vi "Micrometer Heading v2.vi"() -> ()   [LabVIEW 2024]
uses:
  <vilib>/Utility/miscctls.llb/LVRowAndColumnTypeDef.ctl
  Library/Class/Renishaw-XL80_EMU/Renishaw-XL80_EMU.lvclass
  Library/Class/Renishaw-XL80/Renishaw-XL80.lvclass
  <vilib>/Utility/file.llb/Write Delimited Spreadsheet (string).vi
  <vilib>/Analysis/1siggen.llb/Ramp Pattern by Delta.vi
  <vilib>/Analysis/NI_AALBase.lvlib
panel:
  in  "Table Control Periodic":string[][](table)
  in  "Range":u16(ring)=10 caption="mm/inch" items=["0-25"=10, "0-50"=20]
  out "Periodic Range of Errors":dbl=nan format="%#.8f"
  out "Progressive Range of Errors":dbl=nan format="%#.8f"
  out "error out 2":errorcluster
  in  "Clear Result":bool
  in  "Export to CSV":bool
  in  "Delete Down":bool
  in  "Read Down":bool
  in  "Delete Up":bool
  out "Down Values":dbl[](array[numeric]) caption="Down Value" format="%#.6f"
  in  "Read Up":bool
  out "Backlash":dbl=nan format="%#.8f"
  out "Repeatability":dbl=nan format="%#.8f"
  in  "Calculate Read":bool
  out "Up Values":dbl[](array[numeric]) caption="Up Value" format="%#.6f"
  in  "Nominal":dbl caption="Job No." format="%#.8f"
  out "output cluster":cluster{"nextRow":dbl, "nextColumn":dbl}
  out "Current":T1
  out "ScanCode":i16
  in  "Table Control Progressive":string[][](table)
  out "Signal":dbl(slide) scale=0.0..31.0
  in  "sign_mode":bool
  out "Zero Value":dbl format="%_8f"
  out "Mat Temp":dbl[](array[numeric]) caption="Mat Temp(°C)"
  out "Air Temp":dbl caption="Air Temp(°C)"
  in  "Reset":bool
  in  "Connect":bool
  in  "Zero":bool
  out "Serial Number":string caption="Laser Device ID"
  out "Connected":bool
  in  "Precision":u16(ring)=4 items=["0 digit", "1 digit", "2 digits", "3 digits", "4 digits", "5 digits", "6 digits"]
  in  "Unit":u16(ring) caption="mm/inch" items=["mm", "inch"]
  out "Measurement":dbl format="%.4f"
  in  "Description":string
  in  "Manufacturer":string
  in  "Ref equipment ID":string
  in  "Model No.":string
  in  "S/No. or ID":string
  in  "Job No.":string
  out "uncalibrated":dbl
  out "error out":errorcluster
  in  "error IO":errorcluster
  # "Read Value"
  # "Repeatability & Backlash"
  # "Job Info"
  # "DUT Info"
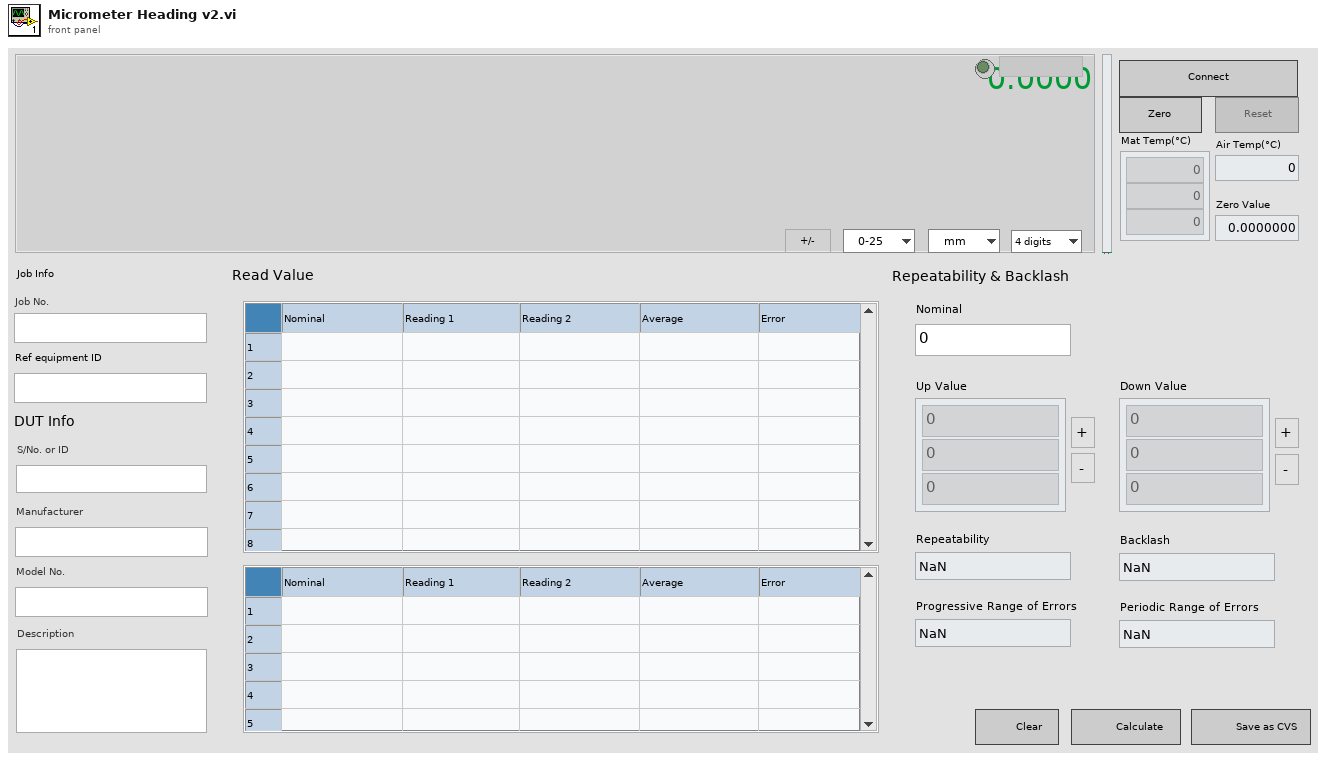
[diagram p1: front panel]
types:
  T1 = typedef "LVRowAndColumnTypeDef.ctl" = cluster{"Row":i32, "Column":i32}
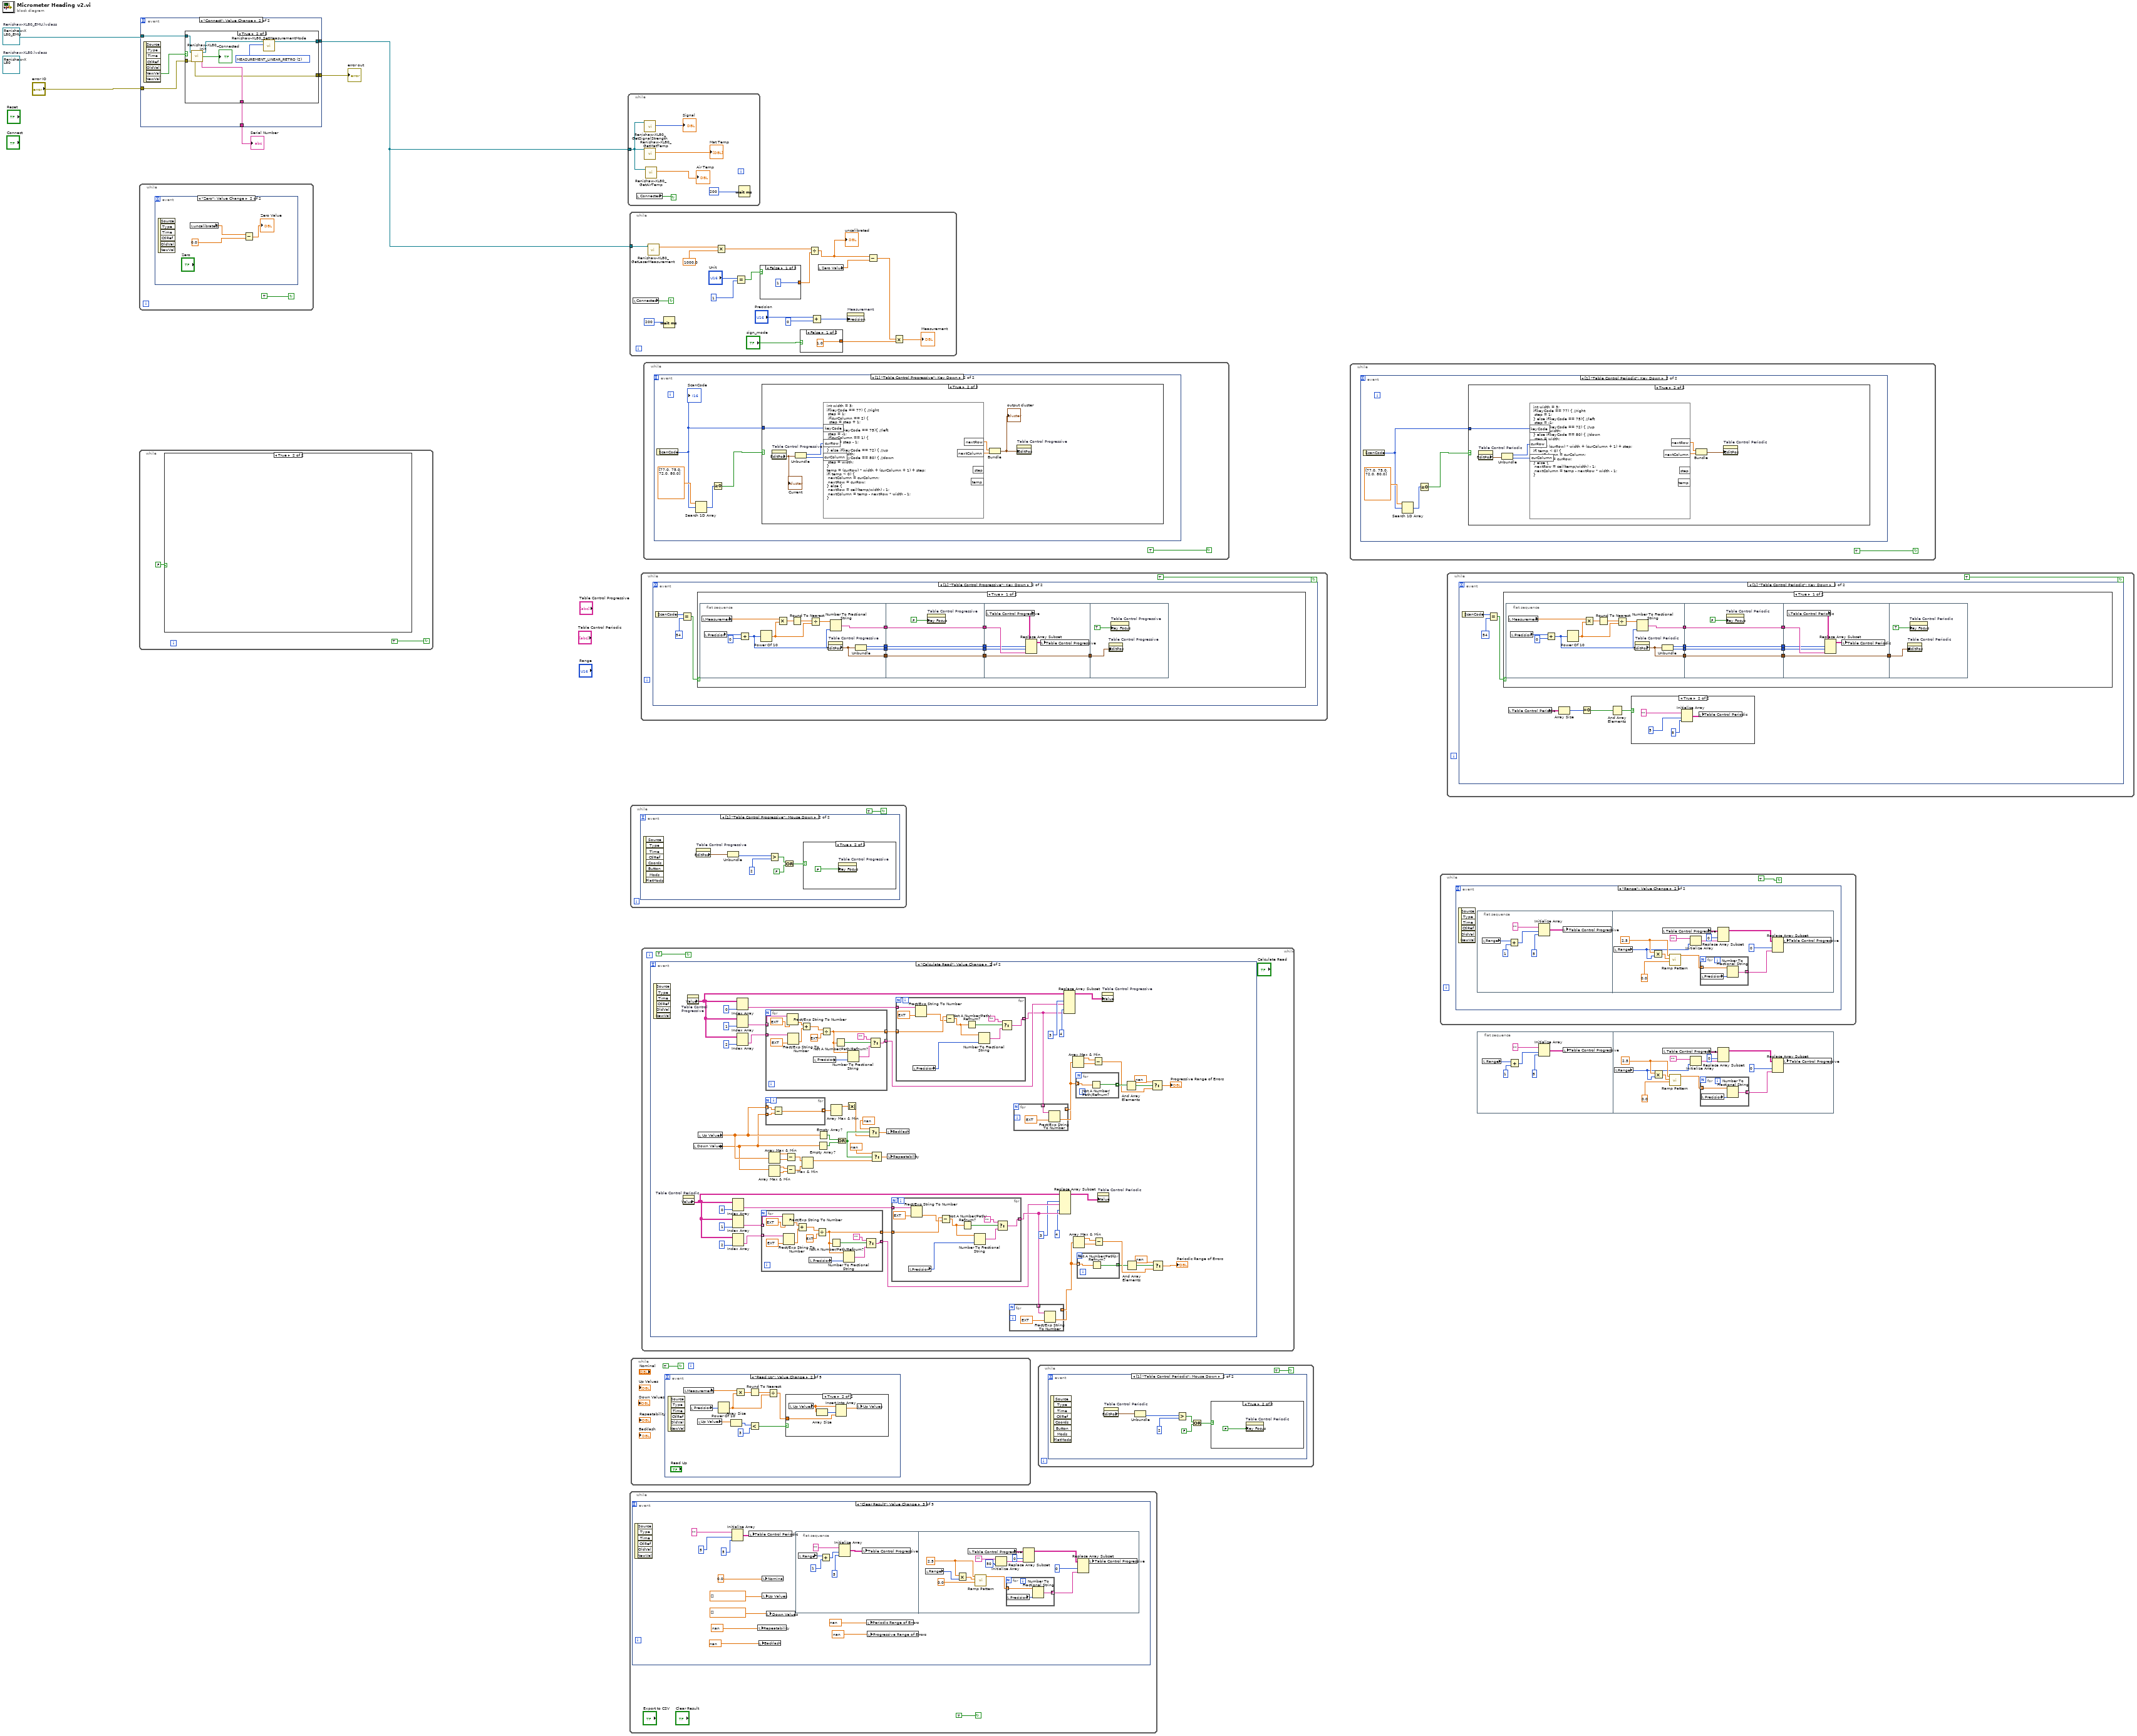
[diagram p0: block diagram]
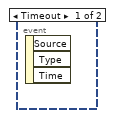
[diagram p2: hidden frame]
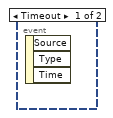
[diagram p4: hidden frame]
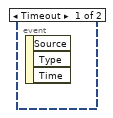
[diagram p6: hidden frame]
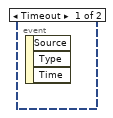
[diagram p9: hidden frame]
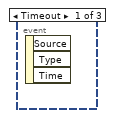
[diagram p10: hidden frame]
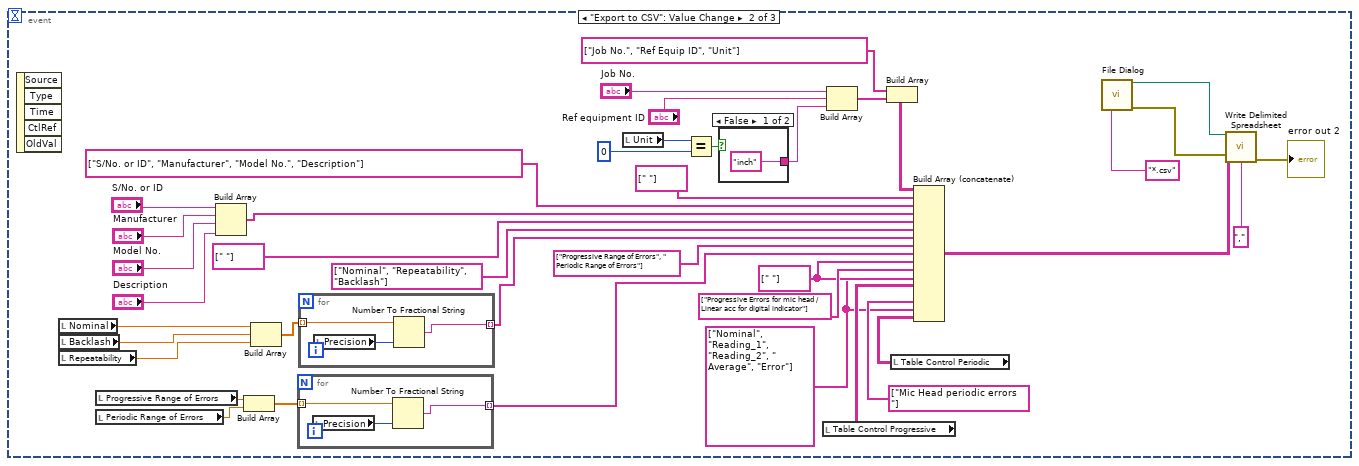
[diagram p11: hidden frame]
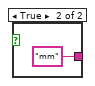
[diagram p12: hidden frame]
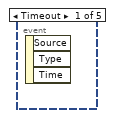
[diagram p13: hidden frame]
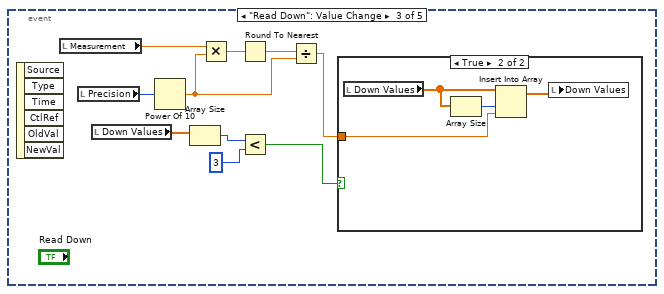
[diagram p15: hidden frame]
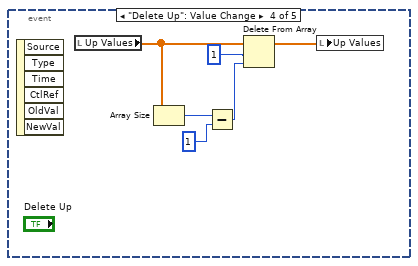
[diagram p17: hidden frame]
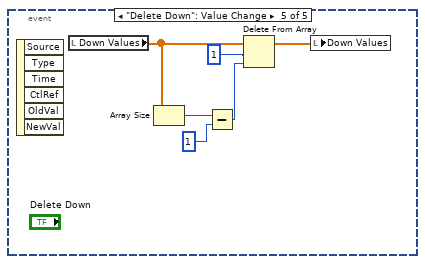
[diagram p18: hidden frame]
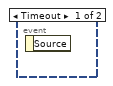
[diagram p19: hidden frame]
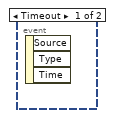
[diagram p20: hidden frame]
diagram:
  w1 = refnum<class "Renishaw-XL80_EMU.lvclass"> refnum  # Renishaw-XL80_EMU.lvclass
  (unwired) refnum<class "Renishaw-XL80.lvclass"> refnum  # Renishaw-XL80.lvclass
  n1 = while {
    stop <- TRUE continue-if-true
    n2 = case shown="True" FALSE {
      frame False {
      }
      frame True {
      }
    }
  }
  n3 = while {
    stop <- TRUE continue-if-true
    n4 = event shown="[1] \"Zero\": Value Change" {
      selector: _ -> [_ _]
      dyn-events: _ -> [_ _]
      timeout: _ -> [_ _]
      event Timeout {
        n5 = event-data() -> ()  [unwired: 1 in, 3 out]
      }
      event "Zero": Value Change {
        n6 = event-data() -> ()  [unwired: 1 in, 6 out]
        n7 = local read "uncalibrated"() -> (w11:dbl)
        n8 = Subtract(x=w11, y=0.0) -> (x-y=→"Zero Value":dbl)
      }
    }
  }
  n9 = event shown="[1] \"Connect\": Value Change" {
    selector: _ -> [_ _]
    dyn-events: _ -> [_ _]
    timeout: _ -> [_ _]
    tunnel: w1 -> [_ w17]
    tunnel: [_ w16] -> w4
    tunnel: [_ w15] -> w5
    tunnel: "error IO" -> [_ w14]
    tunnel: [_ w13] -> w3
    event Timeout {
      n10 = event-data() -> ()  [unwired: 1 in, 3 out]
    }
    event "Connect": Value Change {
      n11 = event-data() -> ("NewVal"=w12:bool)  [unwired: 1 in, 6 out]
      n12 = case shown="True" w12 {
        tunnel: w17 -> [w22 w30]
        tunnel: ["N/A" ("Serial Number") w29] -> w15
        tunnel: [w21 w24] -> w16
        tunnel: w14 -> [w20 w28]
        tunnel: [w19 w27] -> w13
        frame False {
          n13 = call-dynamic "Renishaw-XL80_Close.vi"("error in (no error)"=w20, "Renishaw-XL80_EMU in"=w22) -> ("error out"=w19:errorcluster, "Renishaw-XL80_EMU out"=w21:refnum<class "Renishaw-XL80_EMU.lvclass">)  [unwired: 8 in]
        }
        frame True {
          w23 = 2 items=["MEASUREMENT_INDETERMINATE", "MEASUREMENT_LINEAR_PLANE", "MEASUREMENT_LINEAR_RETRO", "MEASUREMENT_ANGULAR", "MEASUREMENT_STRAIGHTNESS_SHORT", "MEASUREMENT_STRAIGHTNESS_LONG", "MEASUREMENT_VELOCITY_RETRO"] ("MeasurementMode")
          n14 = call-dynamic "Renishaw-XL80_Init.vi"("error in (no error)"=w28, "Renishaw-XL80_EMU in"=w30) -> ("error out"=w27:errorcluster, "Serial Number"=w29:string, "Connect"=→"Connected":bool, "Renishaw-XL80_EMU out"=w25:refnum<class "Renishaw-XL80_EMU.lvclass">)  [unwired: 6 in]
          n15 = call-dynamic "Renishaw-XL80_SetMeasurementMode.vi"("MeasurementMode"=w23, "Renishaw-XL80_EMU in"=w25) -> ("Renishaw-XL80_EMU out"=w24:refnum<class "Renishaw-XL80_EMU.lvclass">)  [unwired: 8 in, 1 out]
        }
      }
    }
  }
  "error out" <- w3
  "Serial Number" <- w5
  n16 = while {
    tunnel: w4 -> [w32]
    stop <- w33 continue-if-true
    n17 = local read "Connected"() -> (w33:bool)
    n18 = call-dynamic "Renishaw-XL80_GetSignalStrength.vi"("Renishaw-XL80_EMU in"=w32) -> ("Signal Strength"=→"Signal":i16)  [unwired: 8 in, 2 out]
    n19 = call-dynamic "Renishaw-XL80_GetMatTemp.vi"("Renishaw-XL80_EMU in"=w32) -> ("Temperature Array"=→"Mat Temp":dbl[])  [unwired: 7 in, 3 out]
    n20 = call-dynamic "Renishaw-XL80_GetAirTemp.vi"("Renishaw-XL80_EMU in"=w32) -> ("GetAirTemp"=→"Air Temp":dbl)  [unwired: 7 in, 3 out]
    n21 = Wait (ms)(milliseconds to wait=u32 200) -> ()  [unwired: 1 out]
  }
  n22 = while {
    tunnel: w4 -> [w55]
    stop <- w44 continue-if-true
    n23 = local read "Connected"() -> (w44:bool)
    n24 = call-dynamic "Renishaw-XL80_GetLaserMeasurement.vi"("Renishaw-XL80_EMU in"=w55) -> ("GetLaserMeasurement"=w53:dbl)  [unwired: 7 in, 3 out]
    n25 = Wait (ms)(milliseconds to wait=u32 200) -> ()  [unwired: 1 out]
    n26 = Multiply(x=w53, y=1000.0) -> (x*y=w45:dbl)
    n27 = Equal?(x="Unit", y=u16 1) -> (x = y?=w47:bool)
    n28 = case shown="False" w47 {
      tunnel: [1 25.4] -> w46
      frame False {
      }
      frame True {
      }
    }
    n29 = case shown="False" "sign_mode" {
      tunnel: [1.0 -1.0] -> w39
      frame False {
      }
      frame True {
      }
    }
    n30 = Divide(x=w45, y=w46) -> (x/y=w42:dbl)
    "uncalibrated" <- w42
    n31 = Add(x="Precision", y=u16 0) -> (x+y=w41:u16)
    n32 = local read "Zero Value"() -> (w43:dbl)
    n33 = property on="Measurement" class="DigNum (strict)"("Precision"=w41) -> ()  [unwired: 2 in, 2 out]
    n34 = Subtract(x=w42, y=w43) -> (x-y=w38:dbl)
    n35 = Multiply(x=w38, y=w39) -> (x*y=→"Measurement":dbl)
  }
  n36 = while {
    stop <- TRUE continue-if-true
    n37 = event shown="[2] \"Clear Result\": Value Change" {
      selector: _ -> [_ _ _]
      dyn-events: _ -> [_ _ _]
      timeout: _ -> [_ _ _]
      event Timeout {
        n38 = event-data() -> ()  [unwired: 1 in, 3 out]
      }
      event "Export to CSV": Value Change {
        w69 = string[] [" "] ("array")
        w66 = string[] ["Nominal", "Reading_1", "Reading_2", " Average", "Error"]
        n39 = event-data() -> ()  [unwired: 1 in, 5 out]
        n40 = local read "Nominal"() -> (w71:dbl)
        n41 = local read "Backlash"() -> (w84:dbl)
        n42 = local read "Repeatability"() -> (w83:dbl)
        n43 = local read "Progressive Range of Errors"() -> (w64:dbl)
        n44 = local read "Periodic Range of Errors"() -> (w62:dbl)
        n45 = Build Array("S/No. or ID", "Manufacturer", "Model No.", "Description") -> (w73:string[])
        n46 = Build Array(w64, w62) -> (w63:dbl[])
        n47 = Build Array(w71, w84, w83) -> (w82:dbl[])
        n48 = for {
          tunnel: w63 -> [w102] mode=indexing
          tunnel: [w101] -> w61 mode=indexing
          n49 = local read "Precision"() -> (w103:u16)
          n50 = Number To Fractional String(number=w102, precision (6)=w103) -> (F-format string=w101:string)  [unwired: 2 in]
        }
        n51 = for {
          tunnel: w82 -> [w105] mode=indexing
          tunnel: [w104] -> w80 mode=indexing
          n52 = local read "Precision"() -> (w106:u16)
          n53 = Number To Fractional String(number=w105, precision (6)=w106) -> (F-format string=w104:string)  [unwired: 2 in]
        }
        n54 = local read "Unit"() -> (w93:u16)
        n55 = Equal?(x=w93, y=u16 0) -> (x = y?=w91:bool)
        n56 = case shown="False" w91 {
          tunnel: ["inch" "mm"] -> w90
          frame False {
          }
          frame True {
          }
        }
        n57 = local read "Table Control Progressive"() -> (w79:string[][])
        n58 = Build Array("Job No.", "Ref equipment ID", w90) -> (w88:string[])
        n59 = Build Array(string[] ["Job No.", "Ref Equip ID", "Unit"] ("element"), w88) -> (w87:string[][])
        n60 = local read "Table Control Periodic"() -> (w67:string[][])
        n61 = Build Array (concatenate)(w87, string[] [" "] ("array"), string[] ["S/No. or ID", "Manufacturer", "Model No.", "Description"] ("element"), w73, string[] [" "] ("array"), string[] ["Nominal", "Repeatability", "Backlash"] ("element"), w80, string[] ["Progressive Range of Errors", " Periodic Range of Errors"] ("element"), w61, w69, string[] ["Progressive Errors for mic head / Linear acc for digital indicator"] ("element"), w66, w79, w69, string[] ["Mic Head periodic errors "] ("element"), w66, w67) -> (w99:string[][])
        n62 = call "File Dialog"("pattern (all files)"="*.csv") -> ("selected path"=w98:path, "error out"=w95:errorcluster)  [unwired: 11 in, 2 out]
        n63 = call-poly <vilib>:"Write Delimited Spreadsheet.vi"("file path (dialog if empty)"=w98, "2D data"=w99, "error in (no error)"=w95, "delimiter (\\t)"="," ("delimiter (\\t)")) -> ("error out"=→"error out 2":errorcluster)  [unwired: 10 in, 1 out]
      }
      event "Clear Result": Value Change {
        n64 = event-data() -> ()  [unwired: 1 in, 6 out]
        n65 = Initialize Array("", 5 ("dimension size"), 5 ("dimension size")) -> (w119:string[][])
        n66 = local write "Table Control Periodic"(w119) -> ()
        n67 = local write "Repeatability"(nan ("Nominal")) -> ()
        n68 = local write "Backlash"(nan ("Nominal")) -> ()
        n69 = local write "Nominal"(0.0 ("Nominal")) -> ()
        n70 = local write "Up Values"(dbl[] [] ("Up Values")) -> ()
        n71 = local write "Down Values"(dbl[] [] ("Up Values")) -> ()
        n72 = flat-sequence {
          frame #0 {
            n73 = local read "Range"() -> (w121:u16)
            n74 = Add(x=w121, y=u16 1) -> (x+y=w122:u16)
            n75 = Initialize Array("", w122, 5 ("dimension size")) -> (w125:string[][])
            n76 = local write "Table Control Progressive"(w125) -> ()
          }
          frame #1 {
            w126 = 2.5 ("delta")
            n77 = local read "Range"() -> (w127:u16)
            n78 = Multiply(x=w126, y=w127) -> (x*y=w128:dbl)
            n79 = local read "Table Control Progressive"() -> (w134:string[][])
            n80 = call-poly <vilib>:"Ramp Pattern.vi"("start"=0.0, "end"=w128, "delta"=w126) -> ("Ramp Pattern"=w130:dbl[])  [unwired: 6 in, 2 out]
            n81 = Initialize Array("", 50 ("dimension size")) -> (w137:string[])
            n82 = for {
              tunnel: w130 -> [w142] mode=indexing
              tunnel: [w140] -> w132 mode=indexing
              n83 = local read "Precision"() -> (w141:u16)
              n84 = Number To Fractional String(number=w142, precision (6)=w141) -> (F-format string=w140:string)  [unwired: 2 in]
            }
            n85 = Replace Array Subset(array=w134, new element=w137, index (col)=0) -> (w139:string[][])  [unwired: 1 in]
            n86 = Replace Array Subset(array=w139, new element=w132, index (col)=0) -> (w131:string[][])  [unwired: 1 in]
            n87 = local write "Table Control Progressive"(w131) -> ()
          }
        }
        n88 = local write "Periodic Range of Errors"(nan ("Nominal")) -> ()
        n89 = local write "Progressive Range of Errors"(nan ("Nominal")) -> ()
      }
    }
  }
  n90 = while {
    stop <- TRUE continue-if-true
    n91 = event shown="[1] \"Table Control Progressive\": Mouse Down" {
      selector: _ -> [_ _]
      dyn-events: _ -> [_ _]
      timeout: _ -> [_ _]
      event Timeout {
        n92 = event-data() -> ()  [unwired: 1 in, 3 out]
      }
      event "Table Control Progressive": Mouse Down {
        n93 = event-data() -> ()  [unwired: 1 in, 8 out]
        n94 = property on="Table Control Progressive" class="Tbl (strict)"() -> ("EditPos"=w149:T1)  [unwired: 2 in, 2 out]
        n95 = Unbundle(w149) -> ("Column"=w147:i32)  [unwired: 1 out]
        n96 = Greater?(x=w147, y=2) -> (0:w146:bool)
        n97 = Or(x=w146, y=FALSE) -> (x .or. y?=w145:bool)
        n98 = case shown="True" w145 {
          frame False {
          }
          frame True {
            n99 = property on="Table Control Progressive" class="Tbl (strict)"("Key Focus"=FALSE) -> ()  [unwired: 2 in, 2 out]
          }
        }
      }
    }
  }
  n100 = while {
    stop <- TRUE continue-if-true
    n101 = event shown="[1] \"Read Up\": Value Change" {
      selector: _ -> [_ _ _ _ _]
      dyn-events: _ -> [_ _ _ _ _]
      timeout: _ -> [_ _ _ _ _]
      event Timeout {
        n102 = event-data() -> ()  [unwired: 1 in, 3 out]
      }
      event "Read Up": Value Change {
        n103 = event-data() -> ()  [unwired: 1 in, 6 out]
        n104 = local read "Measurement"() -> (w157:dbl)
        n105 = local read "Precision"() -> (w161:u16)
        n106 = local read "Up Values"() -> (w156:dbl[])
        n107 = Power Of 10(x=w161) -> (10^x=w158:dbl)
        n108 = Array Size(array=w156) -> (size(s)=w155:i32)
        n109 = Multiply(x=w157, y=w158) -> (x*y=w160:dbl)
        n110 = Round To Nearest(number=w160) -> (nearest integer value=w159:dbl)
        n111 = Less?(x=w155, y=3) -> (x < y?=w153:bool)
        n112 = Divide(x=w159, y=w158) -> (x/y=w152:dbl)
        n113 = case shown="True" w153 {
          tunnel: w152 -> [_ w165]
          frame False {
          }
          frame True {
            n114 = local read "Up Values"() -> (w164:dbl[])
            n115 = Array Size(array=w164) -> (size(s)=w163:i32)
            n116 = Insert Into Array(array=w164, index=w163, new element=w165) -> (w162:dbl[])
            n117 = local write "Up Values"(w162) -> ()
          }
        }
      }
      event "Read Down": Value Change {
        n118 = event-data() -> ()  [unwired: 1 in, 6 out]
        n119 = local read "Measurement"() -> (w171:dbl)
        n120 = local read "Precision"() -> (w175:u16)
        n121 = local read "Down Values"() -> (w170:dbl[])
        n122 = Power Of 10(x=w175) -> (10^x=w172:dbl)
        n123 = Array Size(array=w170) -> (size(s)=w169:i32)
        n124 = Multiply(x=w171, y=w172) -> (x*y=w174:dbl)
        n125 = Round To Nearest(number=w174) -> (nearest integer value=w173:dbl)
        n126 = Less?(x=w169, y=3) -> (x < y?=w167:bool)
        n127 = Divide(x=w173, y=w172) -> (x/y=w166:dbl)
        n128 = case shown="True" w167 {
          tunnel: w166 -> [_ w179]
          frame False {
          }
          frame True {
            n129 = local read "Down Values"() -> (w178:dbl[])
            n130 = Array Size(array=w178) -> (size(s)=w177:i32)
            n131 = Insert Into Array(array=w178, index=w177, new element=w179) -> (w176:dbl[])
            n132 = local write "Down Values"(w176) -> ()
          }
        }
      }
      event "Delete Up": Value Change {
        n133 = event-data() -> ()  [unwired: 1 in, 6 out]
        n134 = local read "Up Values"() -> (w182:dbl[])
        n135 = Array Size(array=w182) -> (size(s)=w184:i32)
        n136 = Subtract(x=w184, y=1) -> (x-y=w181:i32)
        n137 = Delete From Array(array=w182, length=1, index=w181) -> (array with subset deleted=w180:dbl[])  [unwired: 1 out]
        n138 = local write "Up Values"(w180) -> ()
      }
      event "Delete Down": Value Change {
        n139 = event-data() -> ()  [unwired: 1 in, 6 out]
        n140 = local read "Down Values"() -> (w188:dbl[])
        n141 = Array Size(array=w188) -> (size(s)=w190:i32)
        n142 = Subtract(x=w190, y=1) -> (x-y=w187:i32)
        n143 = Delete From Array(array=w188, length=1, index=w187) -> (array with subset deleted=w186:dbl[])  [unwired: 1 out]
        n144 = local write "Down Values"(w186) -> ()
      }
    }
  }
  n145 = while {
    stop <- TRUE continue-if-true
    n146 = event shown="[1] \"Table Control Progressive\": Key Down" {
      selector: _ -> [_ _]
      dyn-events: _ -> [_ _]
      timeout: _ -> [_ _]
      event Timeout {
        n147 = event-data() -> ()  [unwired: 1 in, 3 out]
      }
      event "Table Control Progressive": Key Down {
        n148 = event-data() -> ("ScanCode"=w193:i16)  [unwired: 1 in]
        n149 = Equal?(x=w193, y=i16 54) -> (x = y?=w194:bool)
        n150 = case shown="True" w194 {
          frame True {
            n151 = flat-sequence {
              tunnel: [w208] -> w204
              tunnel: [w207] -> w201
              tunnel: [w206] -> w199
              tunnel: [w205] -> w196
              tunnel: w204 -> [w221]
              tunnel: [w221] -> w203
              tunnel: [w219] -> w202
              tunnel: w201 -> [w219]
              tunnel: [w218] -> w200
              tunnel: w199 -> [w218]
              tunnel: [w217] -> w197
              tunnel: w196 -> [w217]
              tunnel: w203 -> [w226]
              tunnel: w202 -> [w225]
              tunnel: w200 -> [w224]
              tunnel: [w222] -> w198
              tunnel: w197 -> [w222]
              tunnel: w198 -> [w229]
              frame #0 {
                n152 = local read "Measurement"() -> (w213:dbl)
                n153 = local read "Precision"() -> (w212:u16)
                n154 = Add(x=w212, y=u16 0) -> (x+y=w210:u16)
                n155 = Power Of 10(x=w210) -> (10^x=w216:dbl)
                n156 = Multiply(x=w213, y=w216) -> (x*y=w214:dbl)
                n157 = Round To Nearest(number=w214) -> (nearest integer value=w215:dbl)
                n158 = Divide(x=w215, y=w216) -> (x/y=w209:dbl)
                n159 = property on="Table Control Progressive" class="Tbl (strict)"() -> ("EditPos"=w205:T1)  [unwired: 2 in, 2 out]
                n160 = Number To Fractional String(number=w209, precision (6)=w210) -> (F-format string=w208:string)  [unwired: 2 in]
                n161 = Unbundle(w205) -> ("Row"=w207:i32, "Column"=w206:i32)
              }
              frame #1 {
                n162 = property on="Table Control Progressive" class="Tbl (strict)"("Key Focus"=FALSE) -> ()  [unwired: 2 in, 2 out]
              }
              frame #2 {
                n163 = local read "Table Control Progressive"() -> (w227:string[][])
                n164 = Replace Array Subset(array=w227, new element=w226, index (row)=w225, index (col)=w224) -> (w223:string[][])
                n165 = local write "Table Control Progressive"(w223) -> ()
              }
              frame #3 {
                n166 = property on="Table Control Progressive" class="Tbl (strict)"("EditPos"=w229) -> ()  [unwired: 2 in, 2 out]
                n167 = property on="Table Control Progressive" class="Tbl (strict)"("Key Focus"=TRUE) -> ()  [unwired: 2 in, 2 out]
              }
            }
          }
          frame False {
          }
        }
      }
    }
  }
  n168 = while {
    stop <- TRUE continue-if-true
    n169 = event shown="[1] \"Calculate Read\": Value Change" {
      selector: _ -> [_ _]
      dyn-events: _ -> [_ _]
      timeout: _ -> [_ _]
      event Timeout {
        n170 = event-data() -> ()  [unwired: 1 in, 1 out]
      }
      event "Calculate Read": Value Change {
        n171 = event-data() -> ()  [unwired: 1 in, 6 out]
        n172 = property on="Table Control Periodic" class="Tbl (strict)"() -> ("Value"=w264:string[][])  [unwired: 2 in, 2 out]
        n173 = property on="Table Control Progressive" class="Tbl (strict)"() -> ("Value"=w277:string[][])  [unwired: 2 in, 2 out]
        n174 = local read "Down Values"() -> (w254:dbl[])
        n175 = local read "Up Values"() -> (w255:dbl[])
        n176 = Index Array(array=w264, index (col)=0) -> (element=w263:string[])  [unwired: 1 in]
        n177 = Index Array(array=w264, index (col)=1) -> (element=w260:string[])  [unwired: 1 in]
        n178 = Index Array(array=w264, index (col)=2) -> (element=w261:string[])  [unwired: 1 in]
        n179 = Index Array(array=w277, index (col)=0) -> (element=w285:string[])  [unwired: 1 in]
        n180 = Index Array(array=w277, index (col)=1) -> (element=w288:string[])  [unwired: 1 in]
        n181 = Index Array(array=w277, index (col)=2) -> (element=w287:string[])  [unwired: 1 in]
        n182 = for {
          tunnel: w260 -> [w322] mode=indexing
          tunnel: w261 -> [w320] mode=indexing
          tunnel: [w310] -> w262 mode=indexing
          tunnel: [w312] -> w267 mode=indexing
          n183 = Fract/Exp String To Number(string=w322, default (0 dbl)=ext nan ("default (0 DBL)")) -> (number=w318:ext)  [unwired: 2 in, 1 out]
          n184 = Fract/Exp String To Number(string=w320, default (0 dbl)=ext nan ("default (0 DBL)")) -> (number=w317:ext)  [unwired: 2 in, 1 out]
          n185 = Add(x=w318, y=w317) -> (x+y=w316:ext)
          n186 = local read "Precision"() -> (w314:u16)
          n187 = Divide(x=w316, y=ext 2.0) -> (x/y=w310:ext)
          n188 = Not A Number/Path/Refnum?(number/path/refnum=w310) -> (NaN/Path/Refnum?=w313:bool)
          n189 = Number To Fractional String(number=w310, precision (6)=w314) -> (F-format string=w309:string)  [unwired: 2 in]
          n190 = Select(t="", s=w313, f=w309) -> (s? t:f=w312:string)
        }
        n191 = for {
          tunnel: w288 -> [w352] mode=indexing
          tunnel: w287 -> [w350] mode=indexing
          tunnel: [w340] -> w286 mode=indexing
          tunnel: [w342] -> w274 mode=indexing
          n192 = Fract/Exp String To Number(string=w352, default (0 dbl)=ext nan ("default (0 DBL)")) -> (number=w348:ext)  [unwired: 2 in, 1 out]
          n193 = Fract/Exp String To Number(string=w350, default (0 dbl)=ext nan ("default (0 DBL)")) -> (number=w347:ext)  [unwired: 2 in, 1 out]
          n194 = Add(x=w348, y=w347) -> (x+y=w346:ext)
          n195 = local read "Precision"() -> (w344:u16)
          n196 = Divide(x=w346, y=ext 2.0) -> (x/y=w340:ext)
          n197 = Not A Number/Path/Refnum?(number/path/refnum=w340) -> (NaN/Path/Refnum?=w343:bool)
          n198 = Number To Fractional String(number=w340, precision (6)=w344) -> (F-format string=w339:string)  [unwired: 2 in]
          n199 = Select(t="", s=w343, f=w339) -> (s? t:f=w342:string)
        }
        n200 = for {
          tunnel: w255 -> [w328] mode=indexing
          tunnel: w254 -> [w327] mode=indexing
          tunnel: [w326] -> w278 mode=indexing
          n201 = Subtract(x=w328, y=w327) -> (x-y=w326:dbl)
        }
        n202 = Array Max & Min(array=w255) -> (max value=w284:dbl, min value=w283:dbl)  [unwired: 2 out]
        n203 = Array Max & Min(array=w254) -> (max value=w282:dbl, min value=w281:dbl)  [unwired: 2 out]
        n204 = Subtract(x=w284, y=w283) -> (x-y=w256:dbl)
        n205 = Subtract(x=w282, y=w281) -> (x-y=w279:dbl)
        n206 = Max & Min(x=w256, y=w279) -> (max(x,y)=w251:dbl)  [unwired: 1 out]
        n207 = Empty Array?(array=w254) -> (empty?=w252:bool)
        n208 = Empty Array?(array=w255) -> (empty?=w253:bool)
        n209 = Array Max & Min(array=w278) -> (max value=w280:dbl)  [unwired: 3 out]
        n210 = Or(x=w253, y=w252) -> (x .or. y?=w248:bool)
        n211 = Absolute Value(x=w280) -> (abs(x)=w246:dbl)
        n212 = Select(t=nan, s=w248, f=w246) -> (s? t:f=w245:dbl)
        n213 = Select(t=nan, s=w248, f=w251) -> (s? t:f=w249:dbl)
        n214 = local write "Backlash"(w245) -> ()
        n215 = local write "Repeatability"(w249) -> ()
        n216 = for {
          tunnel: w262 -> [w306] mode=indexing
          tunnel: w263 -> [w308] mode=indexing
          tunnel: [w300] -> w269 mode=indexing
          n217 = local read "Precision"() -> (w301:u16)
          n218 = Fract/Exp String To Number(string=w308, default (0 dbl)=ext nan ("default (0 DBL)")) -> (number=w299:ext)  [unwired: 2 in, 1 out]
          n219 = Subtract(x=w306, y=w299) -> (x-y=w302:ext)
          n220 = Not A Number/Path/Refnum?(number/path/refnum=w302) -> (NaN/Path/Refnum?=w303:bool)
          n221 = Number To Fractional String(number=w302, precision (6)=w301) -> (F-format string=w305:string)  [unwired: 2 in]
          n222 = Select(t="", s=w303, f=w305) -> (s? t:f=w300:string)
        }
        n223 = for {
          tunnel: w286 -> [w336] mode=indexing
          tunnel: w285 -> [w338] mode=indexing
          tunnel: [w330] -> w272 mode=indexing
          n224 = local read "Precision"() -> (w331:u16)
          n225 = Fract/Exp String To Number(string=w338, default (0 dbl)=ext nan ("default (0 DBL)")) -> (number=w329:ext)  [unwired: 2 in, 1 out]
          n226 = Subtract(x=w336, y=w329) -> (x-y=w332:ext)
          n227 = Not A Number/Path/Refnum?(number/path/refnum=w332) -> (NaN/Path/Refnum?=w333:bool)
          n228 = Number To Fractional String(number=w332, precision (6)=w331) -> (F-format string=w335:string)  [unwired: 2 in]
          n229 = Select(t="", s=w333, f=w335) -> (s? t:f=w330:string)
        }
        n230 = for {
          tunnel: w269 -> [w298] mode=indexing
          tunnel: [w297] -> w232 mode=indexing
          n231 = Fract/Exp String To Number(string=w298, default (0 dbl)=ext nan ("default (0 DBL)")) -> (number=w297:ext)  [unwired: 2 in, 1 out]
        }
        n232 = for {
          tunnel: w272 -> [w325] mode=indexing
          tunnel: [w324] -> w244 mode=indexing
          n233 = Fract/Exp String To Number(string=w325, default (0 dbl)=ext nan ("default (0 DBL)")) -> (number=w324:ext)  [unwired: 2 in, 1 out]
        }
        n234 = Replace Array Subset(array=w264, new element #1=w267, index (col) #1=3 ("index (col)"), new element #2=w269, index (col) #2=4 ("index (col)")) -> (w265:string[][])  [unwired: 2 in]
        n235 = Replace Array Subset(array=w277, new element #1=w274, index (col) #1=3 ("index (col)"), new element #2=w272, index (col) #2=4 ("index (col)")) -> (w276:string[][])  [unwired: 2 in]
        n236 = Array Max & Min(array=w244) -> (max value=w271:ext, min value=w270:ext)  [unwired: 2 out]
        n237 = Array Max & Min(array=w232) -> (max value=w233:ext, min value=w234:ext)  [unwired: 2 out]
        n238 = for {
          tunnel: w244 -> [w294] mode=indexing
          tunnel: [w295] -> w243 mode=indexing
          n239 = Not A Number/Path/Refnum?(number/path/refnum=w294) -> (NaN/Path/Refnum?=w295:bool)
        }
        n240 = for {
          tunnel: w232 -> [w293] mode=indexing
          tunnel: [w292] -> w235 mode=indexing
          n241 = Not A Number/Path/Refnum?(number/path/refnum=w293) -> (NaN/Path/Refnum?=w292:bool)
        }
        n242 = Subtract(x=w271, y=w270) -> (x-y=w240:ext)
        n243 = Subtract(x=w233, y=w234) -> (x-y=w238:ext)
        n244 = property on="Table Control Periodic" class="Tbl (strict)"("Value"=w265) -> ()  [unwired: 2 in, 2 out]
        n245 = property on="Table Control Progressive" class="Tbl (strict)"("Value"=w276) -> ()  [unwired: 2 in, 2 out]
        n246 = And Array Elements(Boolean array=w243) -> (logical AND=w242:bool)
        n247 = And Array Elements(Boolean array=w235) -> (logical AND=w236:bool)
        n248 = Select(t=nan, s=w242, f=w240) -> (s? t:f=→"Progressive Range of Errors":ext)
        n249 = Select(t=nan, s=w236, f=w238) -> (s? t:f=→"Periodic Range of Errors":ext)
      }
    }
  }
  n250 = while {
    stop <- TRUE continue-if-true
    n251 = event shown="[1] \"Table Control Progressive\": Key Down" {
      selector: _ -> [_ _]
      dyn-events: _ -> [_ _]
      timeout: _ -> [_ _]
      event Timeout {
        n252 = event-data() -> ()  [unwired: 1 in, 3 out]
      }
      event "Table Control Progressive": Key Down {
        n253 = event-data() -> ("ScanCode"=w354:i16)  [unwired: 1 in]
        "ScanCode" <- w354
        n254 = Search 1D Array(1D array=dbl[] [77.0, 75.0, 72.0, 80.0], element=w354) -> (index of element=w356:i32)  [unwired: 1 in]
        n255 = Greater Or Equal To 0?(x=w356) -> (x >= 0?=w355:bool)
        n256 = case shown="True" w355 {
          tunnel: w354 -> [_ w364]
          frame False {
          }
          frame True {
            n257 = property on="Table Control Progressive" class="Tbl (strict)"() -> ("EditPos"=w359:T1)  [unwired: 2 in, 2 out]
            "Current" <- w359
            n258 = Unbundle(w359) -> ("Row"=w363:i32, "Column"=w362:i32)
            n259 = formula code="int width = 3;\nif(keyCode == 77) { //right\n\tstep = 1;\n\tif(curColumn == 2) {\n\t\tstep = step + 1;\n\t}\n} else if(keyCode == 75){ //left\n\tstep = -1;\n\tif(curColumn == 1) {\n\t\tstep = step - 1;\n\t}\n} else if(keyCode == 72) { //up\n\tstep = -width;\n} else if(keyCode == 80) { //down\n\tstep = width;\n}\ntemp = (curRow) * width + (curColumn + 1) + step;\nif( temp < 0) {\n\tnextColumn = curColumn;\n\tnextRow = curRow;\n} else {\n\tnextRow = ceil(temp/width) - 1;\n\tnextColumn = temp - nextRow * width - 1;\n}"("keyCode"=w364, "curRow"=w363, "curColumn"=w362) -> ("nextRow"=w361:dbl, "nextColumn"=w360:dbl)  [unwired: 2 out]
            n260 = Bundle("nextRow"=w361, "nextColumn"=w360) -> (w358:cluster{"nextRow":dbl, "nextColumn":dbl})  [unwired: 1 in]
            "output cluster" <- w358
            n261 = property on="Table Control Progressive" class="Tbl (strict)"("EditPos"=w358) -> ()  [unwired: 2 in, 2 out]
          }
        }
      }
    }
  }
  n262 = while {
    stop <- TRUE continue-if-true
    n263 = event shown="[1] \"Table Control Periodic\": Mouse Down" {
      selector: _ -> [_ _]
      dyn-events: _ -> [_ _]
      timeout: _ -> [_ _]
      event Timeout {
        n264 = event-data() -> ()  [unwired: 1 in, 3 out]
      }
      event "Table Control Periodic": Mouse Down {
        n265 = event-data() -> ()  [unwired: 1 in, 8 out]
        n266 = property on="Table Control Periodic" class="Tbl (strict)"() -> ("EditPos"=w371:T1)  [unwired: 2 in, 2 out]
        n267 = Unbundle(w371) -> ("Column"=w369:i32)  [unwired: 1 out]
        n268 = Greater?(x=w369, y=2) -> (0:w368:bool)
        n269 = Or(x=w368, y=FALSE) -> (x .or. y?=w367:bool)
        n270 = case shown="True" w367 {
          frame False {
          }
          frame True {
            n271 = property on="Table Control Periodic" class="Tbl (strict)"("Key Focus"=FALSE) -> ()  [unwired: 2 in, 2 out]
          }
        }
      }
    }
  }
  n272 = while {
    stop <- TRUE continue-if-true
    n273 = event shown="[1] \"Table Control Periodic\": Key Down" {
      selector: _ -> [_ _]
      dyn-events: _ -> [_ _]
      timeout: _ -> [_ _]
      event Timeout {
        n274 = event-data() -> ()  [unwired: 1 in, 3 out]
      }
      event "Table Control Periodic": Key Down {
        n275 = event-data() -> ("ScanCode"=w374:i16)  [unwired: 1 in]
        n276 = Search 1D Array(1D array=dbl[] [77.0, 75.0, 72.0, 80.0], element=w374) -> (index of element=w376:i32)  [unwired: 1 in]
        n277 = Greater Or Equal To 0?(x=w376) -> (x >= 0?=w375:bool)
        n278 = case shown="True" w375 {
          tunnel: w374 -> [_ w384]
          frame False {
          }
          frame True {
            n279 = property on="Table Control Periodic" class="Tbl (strict)"() -> ("EditPos"=w379:T1)  [unwired: 2 in, 2 out]
            n280 = Unbundle(w379) -> ("Row"=w383:i32, "Column"=w382:i32)
            n281 = formula code="int width = 3;\nif(keyCode == 77) { //right\n\tstep = 1;\n} else if(keyCode == 75){ //left\n\tstep = -1;\n} else if(keyCode == 72) { //up\n\tstep = -width;\n} else if(keyCode == 80) { //down\n\tstep = width;\n}\ntemp = (curRow) * width + (curColumn + 1) + step;\nif( temp < 0) {\n\tnextColumn = curColumn;\n\tnextRow = curRow;\n} else {\n\tnextRow = ceil(temp/width) - 1;\n\tnextColumn = temp - nextRow * width - 1;\n}"("keyCode"=w384, "curRow"=w383, "curColumn"=w382) -> ("nextRow"=w381:dbl, "nextColumn"=w380:dbl)  [unwired: 2 out]
            n282 = Bundle("nextRow"=w381, "nextColumn"=w380) -> (w378:cluster{"nextRow":dbl, "nextColumn":dbl})  [unwired: 1 in]
            n283 = property on="Table Control Periodic" class="Tbl (strict)"("EditPos"=w378) -> ()  [unwired: 2 in, 2 out]
          }
        }
      }
    }
  }
  n284 = while {
    stop <- TRUE continue-if-true
    n285 = event shown="[1] \"Range\": Value Change" {
      selector: _ -> [_ _]
      dyn-events: _ -> [_ _]
      timeout: _ -> [_ _]
      event Timeout {
        n286 = event-data() -> ()  [unwired: 1 in, 3 out]
      }
      event "Range": Value Change {
        n287 = event-data() -> ()  [unwired: 1 in, 6 out]
        n288 = flat-sequence {
          frame #0 {
            n289 = local read "Range"() -> (w388:u16)
            n290 = Add(x=w388, y=u16 1) -> (x+y=w386:u16)
            n291 = Initialize Array("", w386, 5 ("dimension size")) -> (w391:string[][])
            n292 = local write "Table Control Progressive"(w391) -> ()
          }
          frame #1 {
            w394 = 2.5 ("delta")
            n293 = local read "Range"() -> (w393:u16)
            n294 = Multiply(x=w394, y=w393) -> (x*y=w392:dbl)
            n295 = local read "Table Control Progressive"() -> (w400:string[][])
            n296 = call-poly <vilib>:"Ramp Pattern.vi"("start"=0.0, "end"=w392, "delta"=w394) -> ("Ramp Pattern"=w396:dbl[])  [unwired: 6 in, 2 out]
            n297 = Initialize Array("", w393) -> (w402:string[])
            n298 = for {
              tunnel: w396 -> [w407] mode=indexing
              tunnel: [w405] -> w398 mode=indexing
              n299 = local read "Precision"() -> (w406:u16)
              n300 = Number To Fractional String(number=w407, precision (6)=w406) -> (F-format string=w405:string)  [unwired: 2 in]
            }
            n301 = Replace Array Subset(array=w400, new element=w402, index (col)=0) -> (w404:string[][])  [unwired: 1 in]
            n302 = Replace Array Subset(array=w404, new element=w398, index (col)=0) -> (w397:string[][])  [unwired: 1 in]
            n303 = local write "Table Control Progressive"(w397) -> ()
          }
        }
      }
    }
  }
  n304 = while {
    stop <- TRUE continue-if-true
    n305 = event shown="[1] \"Table Control Periodic\": Key Down" {
      selector: _ -> [_ _]
      dyn-events: _ -> [_ _]
      timeout: _ -> [_ _]
      event Timeout {
        n306 = event-data() -> ()  [unwired: 1 in, 3 out]
      }
      event "Table Control Periodic": Key Down {
        n307 = event-data() -> ("ScanCode"=w409:i16)  [unwired: 1 in]
        n308 = Equal?(x=w409, y=i16 54) -> (x = y?=w414:bool)
        n309 = case shown="True" w414 {
          frame True {
            n310 = flat-sequence {
              tunnel: [w432] -> w428
              tunnel: [w431] -> w425
              tunnel: [w430] -> w423
              tunnel: [w429] -> w420
              tunnel: w428 -> [w445]
              tunnel: [w445] -> w427
              tunnel: [w443] -> w426
              tunnel: w425 -> [w443]
              tunnel: [w442] -> w424
              tunnel: w423 -> [w442]
              tunnel: [w441] -> w421
              tunnel: w420 -> [w441]
              tunnel: w427 -> [w450]
              tunnel: w426 -> [w449]
              tunnel: w424 -> [w448]
              tunnel: [w446] -> w422
              tunnel: w421 -> [w446]
              tunnel: w422 -> [w453]
              frame #0 {
                n311 = local read "Measurement"() -> (w437:dbl)
                n312 = local read "Precision"() -> (w436:u16)
                n313 = Add(x=w436, y=u16 0) -> (x+y=w434:u16)
                n314 = Power Of 10(x=w434) -> (10^x=w440:dbl)
                n315 = Multiply(x=w437, y=w440) -> (x*y=w438:dbl)
                n316 = Round To Nearest(number=w438) -> (nearest integer value=w439:dbl)
                n317 = Divide(x=w439, y=w440) -> (x/y=w433:dbl)
                n318 = property on="Table Control Periodic" class="Tbl (strict)"() -> ("EditPos"=w429:T1)  [unwired: 2 in, 2 out]
                n319 = Number To Fractional String(number=w433, precision (6)=w434) -> (F-format string=w432:string)  [unwired: 2 in]
                n320 = Unbundle(w429) -> ("Row"=w431:i32, "Column"=w430:i32)
              }
              frame #1 {
                n321 = property on="Table Control Periodic" class="Tbl (strict)"("Key Focus"=FALSE) -> ()  [unwired: 2 in, 2 out]
              }
              frame #2 {
                n322 = local read "Table Control Periodic"() -> (w451:string[][])
                n323 = Replace Array Subset(array=w451, new element=w450, index (row)=w449, index (col)=w448) -> (w447:string[][])
                n324 = local write "Table Control Periodic"(w447) -> ()
              }
              frame #3 {
                n325 = property on="Table Control Periodic" class="Tbl (strict)"("EditPos"=w453) -> ()  [unwired: 2 in, 2 out]
                n326 = property on="Table Control Periodic" class="Tbl (strict)"("Key Focus"=TRUE) -> ()  [unwired: 2 in, 2 out]
              }
            }
          }
          frame False {
          }
        }
        n327 = local read "Table Control Periodic"() -> (w410:string[][])
        n328 = Array Size(array=w410) -> (size(s)=w411:i32[])
        n329 = Equal To 0?(x=w411) -> (x = 0?=w412:bool[])
        n330 = And Array Elements(Boolean array=w412) -> (logical AND=w413:bool)
        n331 = case shown="True" w413 {
          frame False {
          }
          frame True {
            n332 = Initialize Array("", 5 ("dimension size"), 5 ("dimension size")) -> (w419:string[][])
            n333 = local write "Table Control Periodic"(w419) -> ()
          }
        }
      }
    }
  }
  n334 = flat-sequence {
    frame #0 {
      n335 = local read "Range"() -> (w456:u16)
      n336 = Add(x=w456, y=u16 1) -> (x+y=w454:u16)
      n337 = Initialize Array("", w454, 5 ("dimension size")) -> (w459:string[][])
      n338 = local write "Table Control Progressive"(w459) -> ()
    }
    frame #1 {
      w462 = 2.5 ("delta")
      n339 = local read "Range"() -> (w461:u16)
      n340 = Multiply(x=w462, y=w461) -> (x*y=w460:dbl)
      n341 = local read "Table Control Progressive"() -> (w468:string[][])
      n342 = call-poly <vilib>:"Ramp Pattern.vi"("start"=0.0, "end"=w460, "delta"=w462) -> ("Ramp Pattern"=w464:dbl[])  [unwired: 6 in, 2 out]
      n343 = Initialize Array("", w461) -> (w470:string[])
      n344 = for {
        tunnel: w464 -> [w475] mode=indexing
        tunnel: [w473] -> w466 mode=indexing
        n345 = local read "Precision"() -> (w474:u16)
        n346 = Number To Fractional String(number=w475, precision (6)=w474) -> (F-format string=w473:string)  [unwired: 2 in]
      }
      n347 = Replace Array Subset(array=w468, new element=w470, index (col)=0) -> (w472:string[][])  [unwired: 1 in]
      n348 = Replace Array Subset(array=w472, new element=w466, index (col)=0) -> (w465:string[][])  [unwired: 1 in]
      n349 = local write "Table Control Progressive"(w465) -> ()
    }
  }
